vi "Pre-Build Action.vi"(6 "Top Level/Always Included VIs":path[](array[path]), 7 "Main Destination Path":path, 9 "Target Name":string, 10 "Build Specification Name":string, 11 "Project Path":path) -> (0 "error out":errorcluster)   [LabVIEW 2023]
uses:
  <userlib>/_OpenG.lib/file/file.llb/openg_file.lvlib
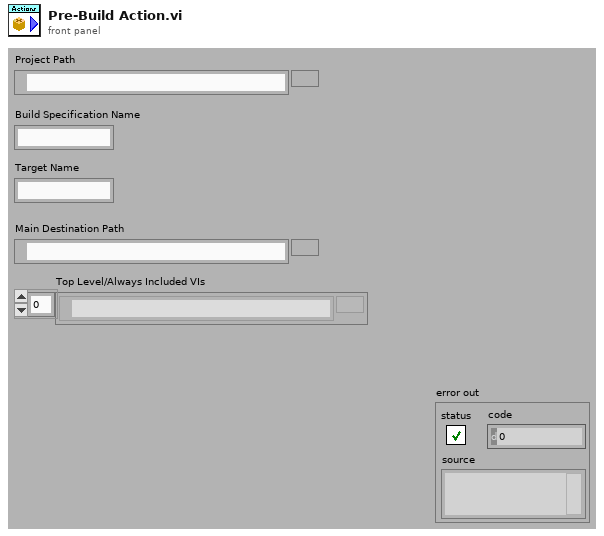
[diagram p1: front panel]
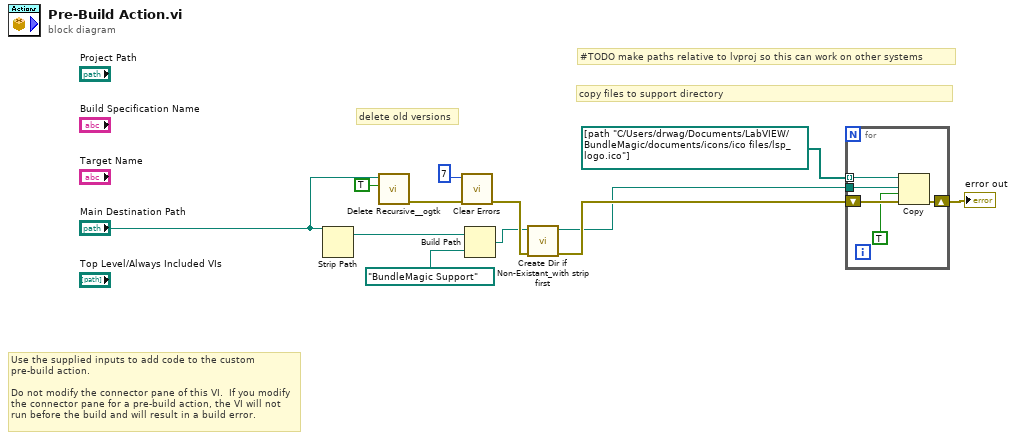
[diagram p0: block diagram]
diagram:
  # "#TODO make paths relative to lvproj so this can work on other systems"
  # "copy files to support directory"
  # "delete old versions"
  # "Use the supplied inputs to add code to the custom pre-build action.\n\nDo not modify the connector pane of this VI.  If you modify the connector pane for a pre-build action, the VI will not run before the build and will result in a build error."
  n1 = Strip Path(path="Main Destination Path") -> (stripped path=w10:path)  [unwired: 1 out]
  n2 = call <userlib>:"Delete Recursive__ogtk.vi"("Recursive? (FALSE)"=TRUE, "Path"="Main Destination Path") -> ("error out"=w9:errorcluster)  [unwired: 8 in, 1 out]
  n3 = call <vilib>:"Clear Errors.vi"("error in (no error)"=w9, "specific error code to clear (0: all)"=7) -> ("error out"=w4:errorcluster)  [unwired: 4 in, 1 out]
  n4 = Build Path(base path=w10, name or relative path=path "BundleMagic Support") -> (appended path=w2:path)
  n5 = call "Create Dir if Non-Existant_with strip first.vi"("error in (no error)"=w4, "Directory Path"=w2) -> ("error out"=w3:errorcluster, "dup Directory Path"=w1:path)  [unwired: 7 in, 1 out]
  n6 = for {
    shift-right: [w16] -> w6
    shift-left: w3 -> [w17]
    tunnel: path[] [path "C:/Users/drwag/Documents/LabVIEW/BundleMagic/documents/icons/ico files/lsp_logo.ico"] ("name or relative path") -> [w15] mode=indexing
    tunnel: w1 -> [w14]
    n7 = Copy(8:w17, 9:TRUE ("overwrite (F)"), 10:w14, 11:w15) -> (0:w16:errorcluster)  [unwired: 1 in, 2 out]
  }
  "error out" <- w6
